vi "UpdateTime.vi"(8 "error in (no error)":errorcluster, 11 "Snake in":refnum<class "Snake.lvclass">) -> (0 "error out":errorcluster, 3 "Snake out":refnum<class "Snake.lvclass">)   [LabVIEW 2019, in "RT_Game.lvlib" / "Snake.lvclass"]
uses:
  Snake.lvclass
  Snake.lvclass/Snake.ctl
  Globals.vi
  RT_Game.lvlib
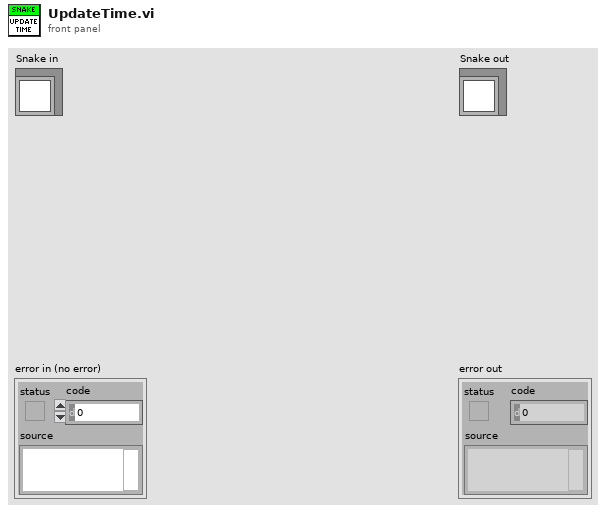
[diagram p1: front panel]
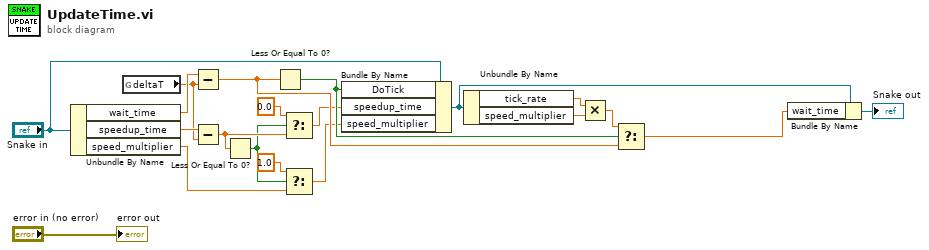
[diagram p0: block diagram]
diagram:
  n1 = Unbundle By Name("Snake in") -> ("wait_time"=w17:dbl, "speedup_time"=w10:dbl, "speed_multiplier"=w5:dbl)
  n2 = global read "Globals.vi" "deltaT"() -> (w9:dbl)
  n3 = Subtract(x=w17, y=w9) -> (x-y=w11:dbl)
  n4 = Subtract(x=w10, y=w9) -> (x-y=w7:dbl)
  n5 = Less Or Equal To 0?(x=w7) -> (x <= 0?=w4:bool)
  n6 = Less Or Equal To 0?(x=w11) -> (x <= 0?=w13:bool)
  n7 = Select(t=0.0, s=w4, f=w7) -> (s? t:f=w8:dbl)
  n8 = Select(t=1.0, s=w4, f=w5) -> (s? t:f=w2:dbl)
  n9 = Bundle By Name(cluster="Snake in", "DoTick"=w13, "speedup_time"=w8, "speed_multiplier"=w2) -> (w16:refnum<class "Snake.lvclass">)
  n10 = Unbundle By Name(w16) -> ("tick_rate"=w15:dbl, "speed_multiplier"=w14:dbl)
  n11 = Multiply(x=w15, y=w14) -> (x*y=w12:dbl)
  n12 = Select(t=w12, s=w13, f=w11) -> (s? t:f=w1:dbl)
  n13 = Bundle By Name(cluster=w16, "wait_time"=w1) -> (→"Snake out":refnum<class "Snake.lvclass">)
  "error out" <- "error in (no error)"
